vi "EncoderTest.vi"() -> ()   [LabVIEW 2015]
uses:
  <vilib>/Rock Robotics/WPI/Counter/WPI_CounterDigitalInputToDigitalSource.vi
  <vilib>/Rock Robotics/SystemInterfaces/DIO/FPGA_DIOChannel.ctl
  <vilib>/Rock Robotics/WPI/Encoder/WPI_EncoderType.ctl
panel:
  in  "stop":bool
  out "Distances":dbl[][](graph)
  out "L Distance":dbl
  out "R Distance":dbl
  in  "Reset":bool
  # "Use this VI to measure Encoder readings"
  # "Move the robot a known distance (tape measure)\nand record the values shown by the encoders"
  # "You can run this code instead of Robot Main,\nbut you will need to push the robot (no motors here)"
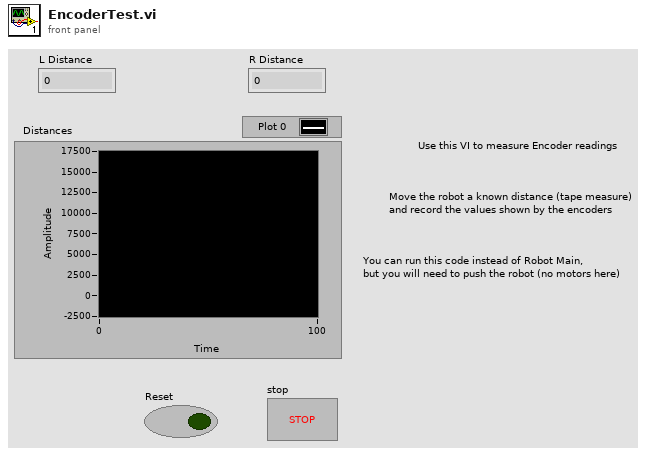
[diagram p1: front panel]
types:
  T1 = typedef "WPI_EncoderDevRef.ctl" = cluster{"DevStatus":errorcluster, "EncoderIndex":T2, "CounterIndex":T3, "DistancePerCount":dbl, "Decoding Type":T4}
  T2 = typedef "FPGA_EncoderIdx.ctl" = enum8{"Enc 0", "Enc 1", "Enc 2", "Enc 3", "Enc 4", "Enc 5", "Enc 6", "Enc 7", "Invalid"}
  T3 = typedef "FPGA_CounterCtrSystemIndex.ctl" = enum8{"Ctr 0", "Ctr 1", "Ctr 2", "Ctr 3", "Ctr 4", "Ctr 5", "Ctr 6", "Ctr 7", "Invalid"}
  T4 = typedef "WPI_EncoderType.ctl" = enum16{"1x", "2x", "4x"}
  T5 = typedef "FPGA_DIOChannel.ctl" = enum8{"DIO 0", "DIO 1", "DIO 2", "DIO 3", "DIO 4", "DIO 5", "DIO 6", "DIO 7", "DIO 8", "DIO 9", "DIO MXP 0", "DIO MXP 1", "DIO MXP 2", "DIO MXP 3", "DIO MXP 4", "DIO MXP 5", "DIO MXP 6", "DIO MXP 7", "DIO MXP 8", "DIO MXP 9", "DIO MXP 10", "DIO MXP 11", "DIO MXP 12", "DIO MXP 13", "DIO MXP 14", "DIO MXP 15", "Invalid"}
  T6 = typedef "WPI_DigitalInputDevRef.ctl" = cluster{"DevStatus":errorcluster, "DIO Channel":T5}
  T7 = typedef "FPGA_CounterEncoderSourceConvertionLVSourceType.ctl" = cluster{"DevStatus":errorcluster, "AnalogTriggerMode?":bool, "DigitalMode":cluster{"DIO Channel":T8}, "AnalogTriggerMode":cluster{"AnalogTriggerIndex":T9, "OutputType":T10}}
  T8 = typedef "FPGA_DIODigitalSourceChannel.ctl" = enum8{"DIO 0", "DIO 1", "DIO 2", "DIO 3", "DIO 4", "DIO 5", "DIO 6", "DIO 7", "DIO 8", "DIO 9", "DIO MXP 0", "DIO MXP 1", "DIO MXP 2", "DIO MXP 3", "DIO MXP 4", "DIO MXP 5", "DIO MXP 6", "DIO MXP 7", "DIO MXP 8", "DIO MXP 9", "DIO MXP 10", "DIO MXP 11", "DIO MXP 12", "DIO MXP 13", "DIO MXP 14", "DIO MXP 15", "Disabled"}
  T9 = typedef "FPGA_AnalogTriggerIndex.ctl" = enum8{"Trig 0", "Trig 1", "Trig 2", "Trig 3", "Trig 4", "Trig 5", "Trig 6", "Trig 7", "Invalid"}
  T10 = typedef "FPGA_AnalogTriggerOutType.ctl" = enum16{"InWindow", "TriggerState", "Rising", "Falling"}
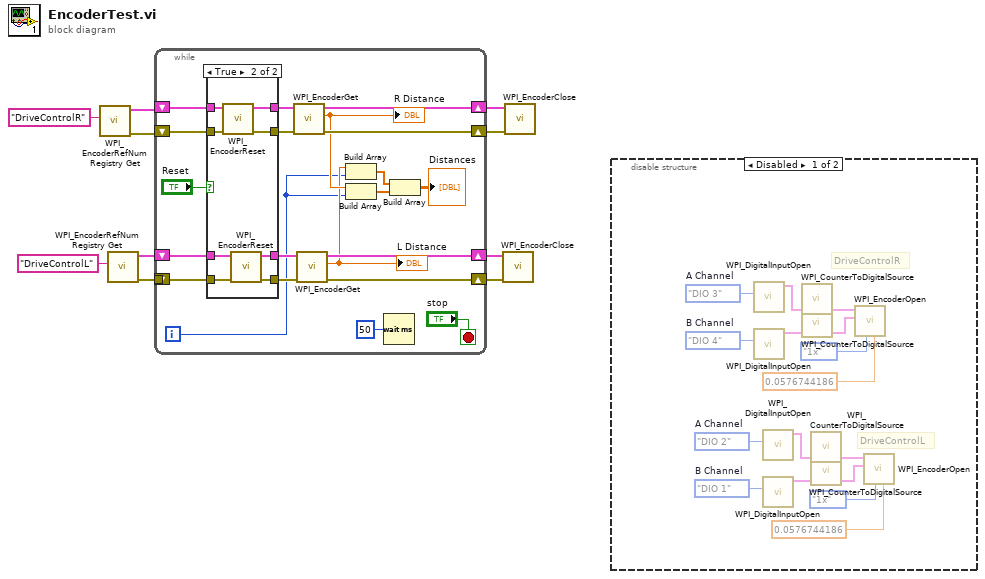
[diagram p0: block diagram]
diagram:
  n1 = call <vilib>:"WPI_EncoderRefNum Registry Get.vi"("refnum name"="DriveControlR") -> ("error out"=w5:errorcluster, "EncoderDevRef"=w6:T1)  [unwired: 9 in]
  n2 = call <vilib>:"WPI_EncoderRefNum Registry Get.vi"("refnum name"="DriveControlL") -> ("error out"=w1:errorcluster, "EncoderDevRef"=w2:T1)  [unwired: 9 in]
  n3 = while {
    tunnel: w1 -> [w25]
    shift-right: [w19] -> w8
    shift-left: _ -> [_]
    shift-right: [w20] -> w7
    shift-left: w2 -> [w27]
    shift-right: [w21] -> w10
    shift-left: w5 -> [w29]
    shift-right: [w22] -> w9
    shift-left: w6 -> [w31]
    i -> [w11]
    stop <- "stop" stop-if-true
    n4 = case shown="True" "Reset" {
      tunnel: w31 -> [w35 w43]
      tunnel: [w35 w42] -> w30
      tunnel: w29 -> [w34 w41]
      tunnel: [w34 w40] -> w28
      tunnel: w27 -> [w33 w39]
      tunnel: [w33 w38] -> w26
      tunnel: w25 -> [w32 w37]
      tunnel: [w32 w36] -> w24
      frame False {
      }
      frame True {
        n5 = call <vilib>:"WPI_EncoderReset.vi"("error in (no error)"=w41, "EncoderDevRef"=w43) -> ("error out"=w40:errorcluster, "EncoderDevRef"=w42:T1)  [unwired: 8 in]
        n6 = call <vilib>:"WPI_EncoderReset.vi"("error in (no error)"=w37, "EncoderDevRef"=w39) -> ("error out"=w36:errorcluster, "EncoderDevRef"=w38:T1)  [unwired: 8 in]
      }
    }
    n7 = call <vilib>:"WPI_EncoderGet.vi"("error in (no error)"=w28, "EncoderDevRef"=w30) -> ("error out"=w21:errorcluster, "Distance"=w13:dbl, "EncoderDevRef"=w22:T1)  [unwired: 4 in, 3 out]
    "R Distance" <- w13
    n8 = call <vilib>:"WPI_EncoderGet.vi"("error in (no error)"=w24, "EncoderDevRef"=w26) -> ("error out"=w19:errorcluster, "Distance"=w12:dbl, "EncoderDevRef"=w20:T1)  [unwired: 4 in, 3 out]
    "L Distance" <- w12
    n9 = Build Array(w12, w11) -> (w16:dbl[])
    n10 = Build Array(w13, w11) -> (w15:dbl[])
    n11 = Wait (ms)(milliseconds to wait=u32 50) -> ()  [unwired: 1 out]
    n12 = Build Array(w16, w15) -> (→"Distances":dbl[][])
  }
  n13 = call <vilib>:"WPI_EncoderClose.vi"("error in (no error)"=w8, "EncoderDevRef"=w7) -> ()  [unwired: 9 in, 1 out]
  n14 = call <vilib>:"WPI_EncoderClose.vi"("error in (no error)"=w10, "EncoderDevRef"=w9) -> ()  [unwired: 9 in, 1 out]
  n15 = disable-structure shown="Disabled" {
    frame Disabled {
      w51 = FPGA_DIOChannel."DIO 4"  # B Channel
      w50 = FPGA_DIOChannel."DIO 3"  # A Channel
      w59 = FPGA_DIOChannel."DIO 1"  # B Channel
      w58 = FPGA_DIOChannel."DIO 2"  # A Channel
      # "DriveControlL"
      # "DriveControlR"
      n16 = call <vilib>:"WPI_DigitalInputOpen.vi"("DIO Channel"=w50) -> ("DigitalInputDevRef"=w47:T6)  [unwired: 1 in, 9 out]
      n17 = call <vilib>:"WPI_DigitalInputOpen.vi"("DIO Channel"=w51) -> ("DigitalInputDevRef"=w48:T6)  [unwired: 1 in, 9 out]
      n18 = call <vilib>:"WPI_DigitalInputOpen.vi"("DIO Channel"=w58) -> ("DigitalInputDevRef"=w55:T6)  [unwired: 1 in, 9 out]
      n19 = call <vilib>:"WPI_DigitalInputOpen.vi"("DIO Channel"=w59) -> ("DigitalInputDevRef"=w56:T6)  [unwired: 1 in, 9 out]
      n20 = call-poly <vilib>:"WPI_CounterToDigitalSource.vi"("DigitalInputDevRef"=w47) -> ("Digital Source"=w46:T7)  [unwired: 6 out]
      n21 = call-poly <vilib>:"WPI_CounterToDigitalSource.vi"("DigitalInputDevRef"=w48) -> ("Digital Source"=w49:T7)  [unwired: 6 out]
      n22 = call-poly <vilib>:"WPI_CounterToDigitalSource.vi"("DigitalInputDevRef"=w55) -> ("Digital Source"=w54:T7)  [unwired: 6 out]
      n23 = call-poly <vilib>:"WPI_CounterToDigitalSource.vi"("DigitalInputDevRef"=w56) -> ("Digital Source"=w57:T7)  [unwired: 6 out]
      n24 = call <vilib>:"WPI_EncoderOpen.vi"("DistancePerCount"=0.0576744186, "Decoding Type"=WPI_EncoderType."1x", "BSource"=w49, "ASource"=w46) -> ()  [unwired: 4 in, 4 out]
      n25 = call <vilib>:"WPI_EncoderOpen.vi"("DistancePerCount"=0.0576744186, "Decoding Type"=WPI_EncoderType."1x", "BSource"=w57, "ASource"=w54) -> ()  [unwired: 4 in, 4 out]
    }
    frame Enabled {
    }
  }
